vi "Read 1.vi"(8 "error in (no error)":errorcluster, 11 "test displayable in":refnum<class "test displayable.lvclass">) -> (0 "error out":errorcluster, 2 "1":dbl, 3 "test displayable out":refnum<class "test displayable.lvclass">)   [LabVIEW 2013, in "test displayable.lvclass"]
uses:
  test displayable.lvclass
  test displayable.lvclass/test displayable.ctl
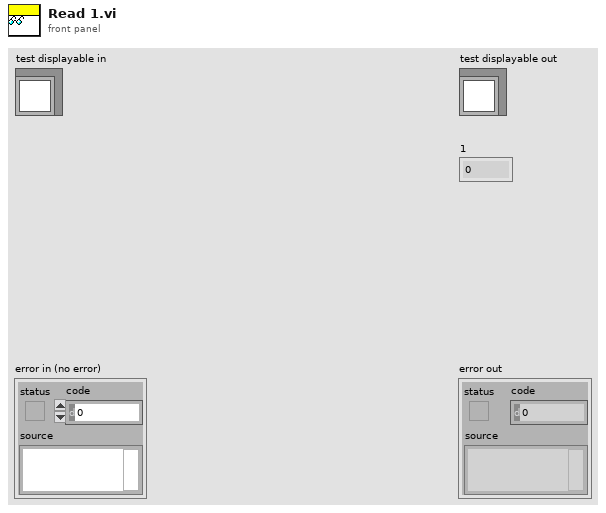
[diagram p1: front panel]
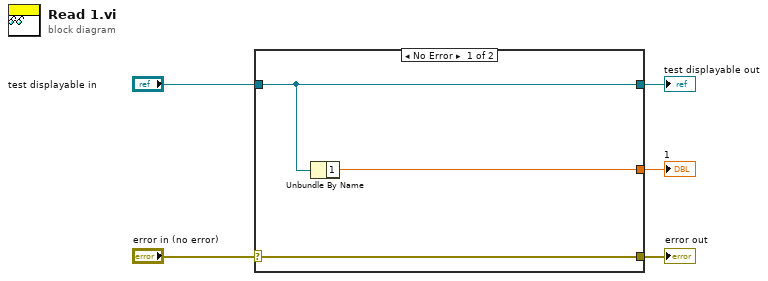
[diagram p0: block diagram]
diagram:
  n1 = case shown="No Error" "error in (no error)" {
    selector: "error in (no error)" -> [w8 w9]
    tunnel: [w8 w9] -> w4
    tunnel: [w7 w10] -> w2
    tunnel: "test displayable in" -> [w7 w10]
    tunnel: [w6 _] -> w1
    frame No Error {
      n2 = Unbundle By Name(w7) -> ("1"=w6:dbl)
    }
    frame Error {
    }
  }
  "error out" <- w4
  "test displayable out" <- w2
  "1" <- w1
